vi "emi_Dialog Init.vi"(1 "Header String(\"\")":string, 5 "Show VI(T)":bool=TRUE, 7 "Use Version info in header(T)":bool=TRUE, 9 "Reinit all controls(F)":bool, 11 "error in":errorcluster, 12 "Center in bottom FP(T)":bool=TRUE, 13 "Set BG Color(T)":bool=TRUE, 14 "Modal(T)":bool=TRUE) -> (15 "error out":errorcluster)   [LabVIEW 2011]
doc: "Initialises a Dialog box. \nNote if initialisation is to performed for the dialog box, it should be done between a hide, and this"
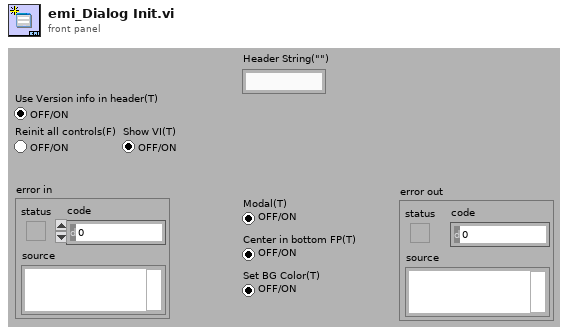
[diagram p1: front panel]
types:
  T1 = enum32{"Invalid", "Default", "Floating", "Floating/Auto-Hide", "Modal"}
  T2 = enum32{"Invalid", "Standard", "Closed", "Hidden", "Minimized", "Maximized"}
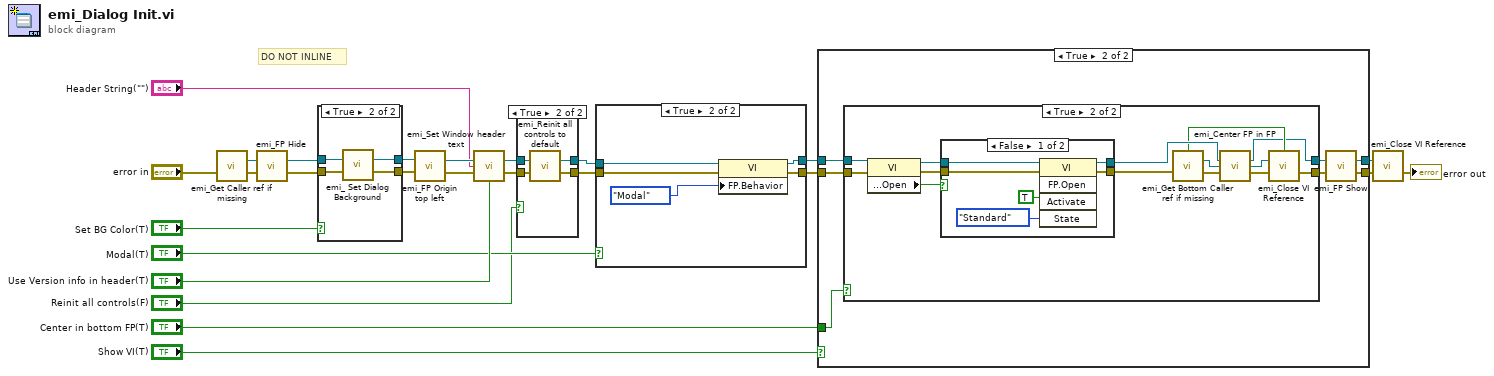
[diagram p0: block diagram]
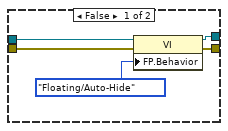
[diagram p6: hidden frame]
diagram:
  # "DO NOT INLINE"
  n1 = call "emi_Get Caller ref if missing.vi"("error in (no error)"="error in") -> ("VI Refnum Out"=w22:refnum<vi>, "error out"=w21:errorcluster)  [unwired: 12 in, 1 out]
  n2 = call "emi_FP Hide.vi"("VI Refnum(This vi)"=w22, "error in (no error)"=w21) -> ("VI Refnum"=w1:refnum<vi>, "error out"=w2:errorcluster)  [unwired: 12 in]
  n3 = case shown="True" "Set BG Color(T)" {
    tunnel: w2 -> [w26 w31]
    tunnel: [w26 w30] -> w20
    tunnel: w1 -> [w27 w29]
    tunnel: [w27 w28] -> w19
    frame False {
    }
    frame True {
      n4 = call "emi_ Set Dialog Background.vi"("VI Refnum(This vi)"=w29, "error in (no error)"=w31) -> ("VI Refnum"=w28:refnum<vi>, "error out"=w30:errorcluster)  [unwired: 12 in]
    }
  }
  n5 = call "emi_FP Origin top left.vi"("VI Refnum(This vi)"=w19, "error in (no error)"=w20) -> ("VI Refnum"=w23:refnum<vi>, "error out"=w24:errorcluster)  [unwired: 12 in]
  n6 = call "emi_Set Window header text.vi"("VI Refnum(This VI)"=w23, "Header String"="Header String(\"\")", "error in (no error)"=w24, "Use Version info(F)"="Use Version info in header(T)") -> ("VI Refnum"=w16:refnum<vi>, "error out"=w15:errorcluster)  [unwired: 10 in]
  n7 = case shown="True" "Reinit all controls(F)" {
    tunnel: w16 -> [w33 w37]
    tunnel: w15 -> [w32 w36]
    tunnel: [w32 w35] -> w12
    tunnel: [w33 w34] -> w11
    frame False {
    }
    frame True {
      n8 = call "emi_Reinit all controls to default.vi"("VI Refnum(This vi)"=w37, "error in (no error)"=w36) -> ("VI Refnum"=w34:refnum<vi>, "error out"=w35:errorcluster)  [unwired: 12 in]
    }
  }
  n9 = case shown="True" "Modal(T)" {
    tunnel: w12 -> [w41 w47]
    tunnel: w11 -> [w39 w46]
    tunnel: [w40 w45] -> w9
    tunnel: [w38 w44] -> w7
    frame False {
      n10 = property class="VI"(reference=w39, error in=w41, "FP.Behavior"=T1."Floating/Auto-Hide" ("Front Panel Window:Behavior")) -> (reference out=w38:refnum<vi>, error out=w40:errorcluster)
    }
    frame True {
      n11 = property class="VI"(reference=w46, error in=w47, "FP.Behavior"=T1."Modal" ("Front Panel Window:Behavior")) -> (reference out=w44:refnum<vi>, error out=w45:errorcluster)
    }
  }
  n12 = case shown="True" "Show VI(T)" {
    tunnel: w9 -> [w48 w53]
    tunnel: [w48 w56] -> w8
    tunnel: w7 -> [w49 w52]
    tunnel: [w49 w55] -> w6
    tunnel: "Center in bottom FP(T)" -> [_ w54]
    frame False {
    }
    frame True {
      n13 = case shown="True" w54 {
        tunnel: w53 -> [w57 w68]
        tunnel: [w57 w72] -> w51
        tunnel: w52 -> [w58 w67]
        tunnel: [w58 w59] -> w50
        frame False {
        }
        frame True {
          n14 = property class="VI"(reference=w67, error in=w68) -> (reference out=w71:refnum<vi>, error out=w70:errorcluster, "Front Panel.Open"=w69:bool)
          n15 = case shown="False" w69 {
            tunnel: w70 -> [w77 w79]
            tunnel: w71 -> [w78 w80]
            tunnel: [w76 w79] -> w66
            tunnel: [w75 w80] -> w65
            frame False {
              n16 = invoke class="VI" method="FP.Open"(reference=w78, error in=w77, "Activate"=TRUE ("Activate?"), "State"=T2."Standard") -> (reference out=w75:refnum<vi>, error out=w76:errorcluster)  [unwired: 1 in, 3 out]
            }
            frame True {
            }
          }
          n17 = call "emi_Get Bottom Caller ref if missing.vi"("error in (no error)"=w66) -> ("Ref Generated"=w60:bool, "VI Refnum Out"=w62:refnum<vi>, "error out"=w64:errorcluster)  [unwired: 12 in]
          n18 = call "emi_Center FP in FP.vi"("VI To position Refnum(This vi)"=w65, "VI Anchor Refnum(Caller)"=w62, "error in (no error)"=w64) -> ("VI to Position Refnum"=w59:refnum<vi>, "VI Anchor Refnum"=w61:refnum<vi>, "error out"=w63:errorcluster)  [unwired: 10 in]
          n19 = call "emi_Close VI Reference.vi"("Close ref?(T)"=w60, "VI Refnum"=w61, "error in (no error)"=w63) -> ("error out"=w72:errorcluster)  [unwired: 11 in, 1 out]
        }
      }
      n20 = call "emi_FP Show.vi"("VI Refnum(This vi)"=w50, "error in (no error)"=w51) -> ("VI Refnum"=w55:refnum<vi>, "error out"=w56:errorcluster)  [unwired: 12 in]
    }
  }
  n21 = call "emi_Close VI Reference.vi"("VI Refnum"=w6, "error in (no error)"=w8) -> ("error out"=→"error out":errorcluster)  [unwired: 12 in, 1 out]
